vi "programa 9.vi"() -> ()   [LabVIEW 2011]
panel:
  in  "on/off Prg":bool
  out "Temp Mínima":dbl
  out "Temp Máxima":dbl
  out "Temp Promedio":dbl
  in  "on/off A/C":bool
  out "A/C on":bool
  in  "Temp Deseada":dbl
  out "Temperatura":i32(slide) scale=0.0..50.0
  # "El programa simula el funcionamiento de un A/C\ndonde se ingresa la temperatura deseada y cada\nvez que la temperatura deseada sea mayor a\n temperatura no se enciende el compresor del\nA/C pero cuando esta sea menor se enciende el compresor\npero este solo puede ocurrir siempre que el A/C este\nencendido, el programa termina solo cuando decidimos\nnosotros terminar"
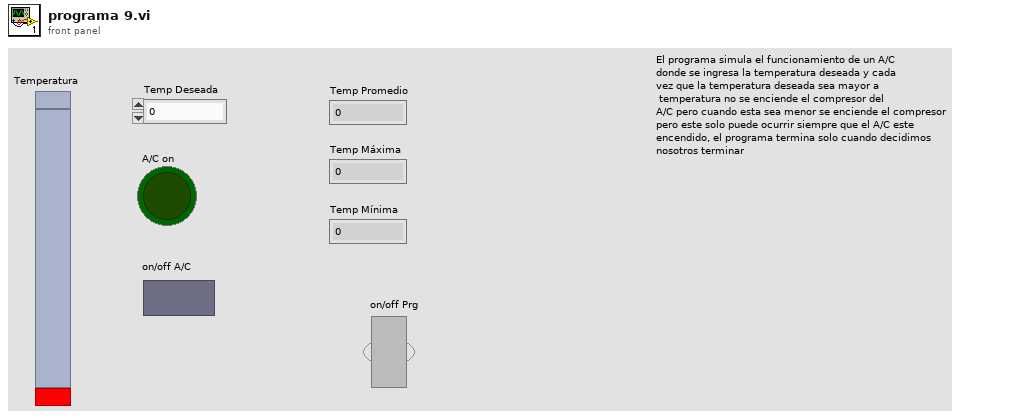
[diagram p1: front panel]
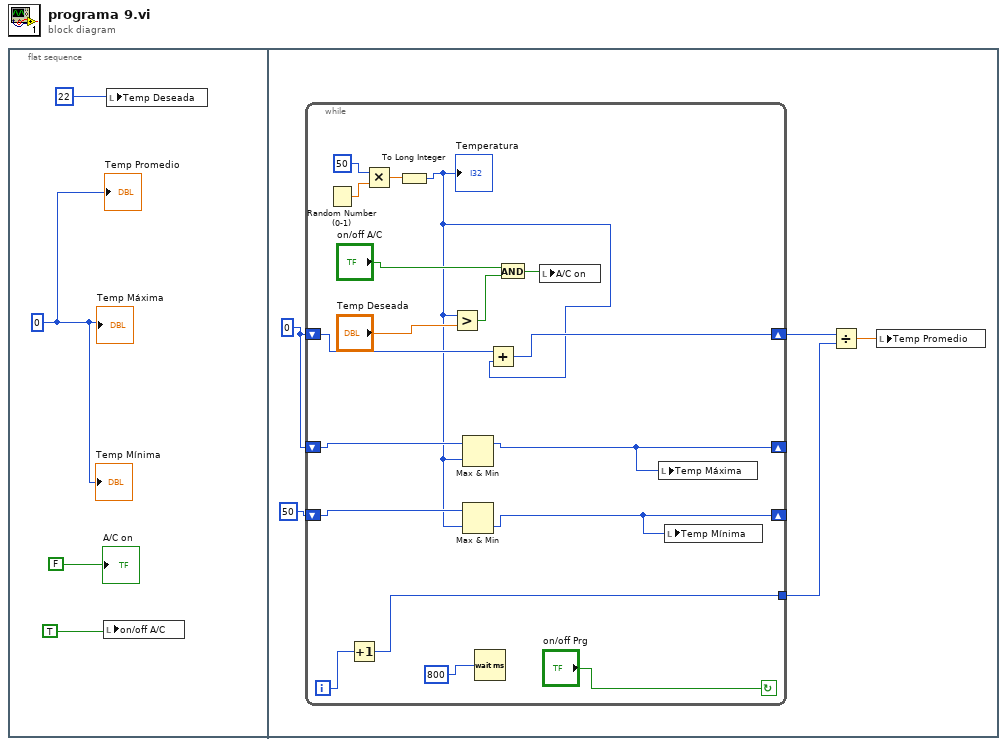
[diagram p0: block diagram]
diagram:
  n1 = flat-sequence {
    frame #0 {
      w4 = 0
      n2 = local write "on/off A/C"(TRUE) -> ()
      n3 = local write "Temp Deseada"(22) -> ()
      "A/C on" <- FALSE
      "Temp Promedio" <- w4
      "Temp Máxima" <- w4
      "Temp Mínima" <- w4
    }
    frame #1 {
      w6 = 0
      n4 = while {
        tunnel: [w17] -> w8
        shift-right: [w15] -> w7
        shift-left: w6 -> [w16]
        shift-right: [w11] -> _
        shift-left: w6 -> [w14]
        shift-right: [w10] -> _
        shift-left: 50 -> [w13]
        i -> [w18]
        stop <- "on/off Prg" continue-if-true
        n5 = Random Number (0-1)() -> (number: 0 to 1=w25:dbl)
        n6 = Increment(x=w18) -> (x+1=w17:i32)
        n7 = Multiply(x=50, y=w25) -> (x*y=w24:dbl)
        n8 = To Long Integer(number=w24) -> (32bit integer=w12:i32)
        "Temperatura" <- w12
        n9 = Greater?(x=w12, y="Temp Deseada") -> (0:w21:bool)
        n10 = Max & Min(x=w14, y=w12) -> (max(x,y)=w11:i32)  [unwired: 1 out]
        n11 = Max & Min(x=w13, y=w12) -> (min(x,y)=w10:i32)  [unwired: 1 out]
        n12 = Wait (ms)(milliseconds to wait=800) -> ()  [unwired: 1 out]
        n13 = Add(x=w16, y=w12) -> (x+y=w15:i32)
        n14 = And(x="on/off A/C", y=w21) -> (x .and. y?=w19:bool)
        n15 = local write "A/C on"(w19) -> ()
        n16 = local write "Temp Máxima"(w11) -> ()
        n17 = local write "Temp Mínima"(w10) -> ()
      }
      n18 = Divide(x=w7, y=w8) -> (x/y=w9:dbl)
      n19 = local write "Temp Promedio"(w9) -> ()
    }
  }
